vi "Format Packet Bytes.vi"(11 "frame data":u8[](array[numeric])) -> (3 "spreadsheet string":string)   [LabVIEW 2025, in "Automotive Ethernet Bus Monitor.lvclass"]
uses:
  Automotive Ethernet Bus Monitor.lvclass
  <vilib>/Utility/error.llb/whitespace.ctl
  <vilib>/Utility/error.llb/Trim Whitespace One-Sided.vi
  Automotive Ethernet Bus Monitor.lvclass/Automotive Ethernet Bus Monitor.ctl
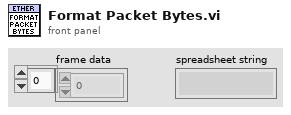
[diagram p1: front panel]
types:
  T1 = typedef "whitespace.ctl" = u16
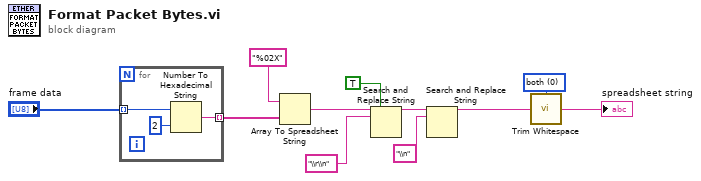
[diagram p0: block diagram]
diagram:
  w1 = T1 0 items=["both", "start of string", "end of string"] ("location (both)")
  n1 = for {
    tunnel: "frame data" -> [w14] mode=indexing
    tunnel: [w13] -> w11 mode=indexing
    n2 = Number To Hexadecimal String(1:i16 2 ("width (-)"), 2:w14) -> (0:w13:string)
  }
  n3 = Array To Spreadsheet String(array=w11, 3:"%02X" ("format string")) -> (spreadsheet string=w8:string)  [unwired: 1 in]
  n4 = Search and Replace String(replace all?=TRUE ("replace all? (F)"), input string=w8, search string="\\r\\n") -> (result string=w5:string)  [unwired: 5 in, 3 out]
  n5 = Search and Replace String(input string=w5, search string="\\n") -> (result string=w3:string)  [unwired: 6 in, 3 out]
  n6 = call <vilib>:"Trim Whitespace.vi"("string"=w3, "location (both)"=w1) -> ("trimmed string"=→"spreadsheet string":string)
